vi "readini2.vi"(4 "error in":errorcluster, 6 "Numeric":i32) -> (0 "error out":errorcluster)   [LabVIEW 2010]
uses:
  Global 2.vi
  <vilib>/Utility/config.llb/NI_LVConfig.lvlib
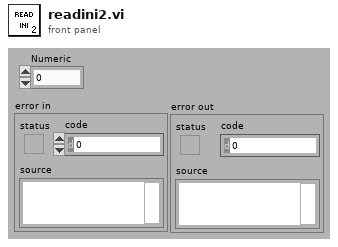
[diagram p1: front panel]
types:
  T1 = typedef "NI_LVConfig.lvlib/Config Data RefNum.ctl" = refnum<k1>
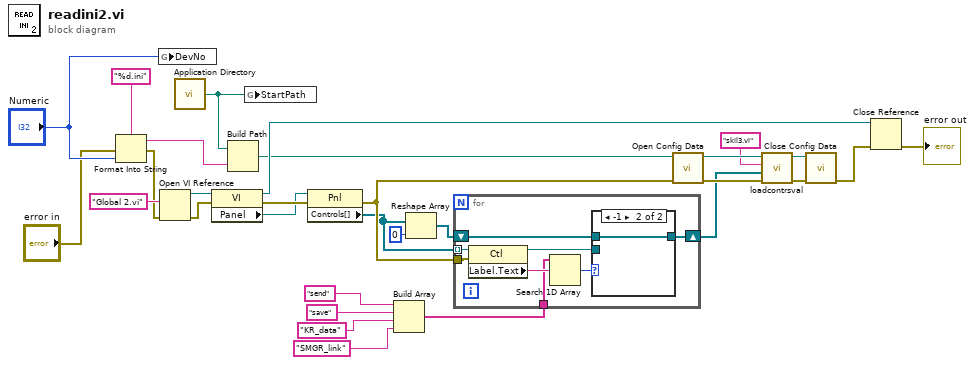
[diagram p0: block diagram]
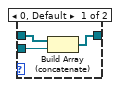
[diagram p2: hidden frame]
diagram:
  n1 = Format Into String(format string="%d.ini" ("string"), error in="error in", "Numeric") -> (resulting string=w28:string, error out=w1:errorcluster)  [unwired: 1 in]
  n2 = global write "Global 2.vi" "DevNo"("Numeric") -> ()
  n3 = Open VI Reference(vi path="Global 2.vi", error in (no error)=w1) -> (vi reference=w6:refnum<vi>, error out=w7:errorcluster)  [unwired: 4 in]
  n4 = call <vilib>:"Application Directory.vi"() -> ("Application Directory"=w3:path)
  n5 = property class="VI"(reference=w6, error in=w7) -> (reference out=w10:refnum<vi>, error out=w9:errorcluster, "Panel"=w8:refnum<vi>)
  n6 = Build Path(base path=w3, name or relative path=w28) -> (appended path=w4:path)
  n7 = global write "Global 2.vi" "StartPath"(w3) -> ()
  n8 = property class="Pnl"(reference=w8, error in=w9) -> (error out=w18:errorcluster, "Controls[]"=w12:refnum<vi>[])  [unwired: 1 out]
  n9 = Build Array("send" ("key"), "save" ("key"), "KR_data" ("key"), "SMGR_link" ("key")) -> (w26:string[])
  n10 = Reshape Array(w12, 0 ("dimension size")) -> (w13:refnum<vi>[])
  n11 = for {
    tunnel: w12 -> [w38] mode=indexing
    tunnel: w18 -> [w34]
    shift-right: [w33] -> w11
    shift-left: w13 -> [w32]
    tunnel: w26 -> [w31]
    n12 = property class="Ctl"(reference=w38, error in=w34) -> (reference out=w35:refnum<vi>, "Label.Text"=w37:string)  [unwired: 1 out]
    n13 = Search 1D Array(1D array=w31, element=w37) -> (index of element=w36:i32)  [unwired: 1 in]
    n14 = case shown="-1" w36 {
      tunnel: w35 -> [w41 _]
      tunnel: [w40 w42] -> w33
      tunnel: w32 -> [w39 w42]
      frame 0, Default {
        n15 = Build Array (concatenate)(w39, w41) -> (w40:refnum<vi>[])
      }
      frame -1 {
      }
    }
  }
  n16 = call <vilib>:"Open Config Data.vi"("error in (no error)"=w18, "configuration file path"=w4) -> ("error out"=w19:errorcluster, "refnum"=w16:T1)  [unwired: 7 in, 1 out]
  n17 = call "loadcontrsval.vi"("error in"=w19, "Array"=w11, "Section"="skil3.vi" ("section"), "refnum in"=w16) -> ("error out"=w20:errorcluster, "refnum out"=w17:T1)  [unwired: 1 in, 1 out]
  n18 = call <vilib>:"Close Config Data.vi"("error in (no error)"=w20, "refnum"=w17) -> ("error out"=w21:errorcluster)  [unwired: 8 in, 1 out]
  n19 = Close Reference(reference=w10, error in (no error)=w21) -> (error out=→"error out":errorcluster)
